vi "DEBUG Simple Node.vi"() -> ()   [LabVIEW 2013]
uses:
  C:/LabQt/LabQt.dll
panel:
  out "str":string
  out "errorCode":i32
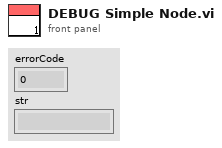
[diagram p1: front panel]
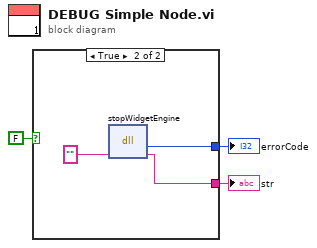
[diagram p0: block diagram]
diagram:
  n1 = case shown="True" FALSE {
    tunnel: [_ w6] -> w3
    tunnel: [_ w4] -> w2
    frame False {
    }
    frame True {
      n2 = dll-call lib="C:/LabQt/LabQt.dll" fn="stopWidgetEngine"("str"="") -> ("errorCode"=w6:i32, "str"=w4:string)  [unwired: 3 in, 2 out]
    }
  }
  "errorCode" <- w3
  "str" <- w2
